vi "Flush Port.vi"(8 "error in (no error)":errorcluster, 10 "Port":T1="Mod6\\Port1", 11 "MPU in":refnum<class "MPU.lvclass">) -> (0 "error out":errorcluster, 3 "MPU out":refnum<class "MPU.lvclass">)   [LabVIEW 2018, in "Modbus_Processing_Unit.lvlib" / "MPU.lvclass"]
uses:
  MPU.lvclass
  PortType.ctl
  <vilib>/rvi/eio/common/nirviEmuTemplateMethod_errors.vi
  <vilib>/eio/EIOMethodNode/EIOMethodNode.xnode
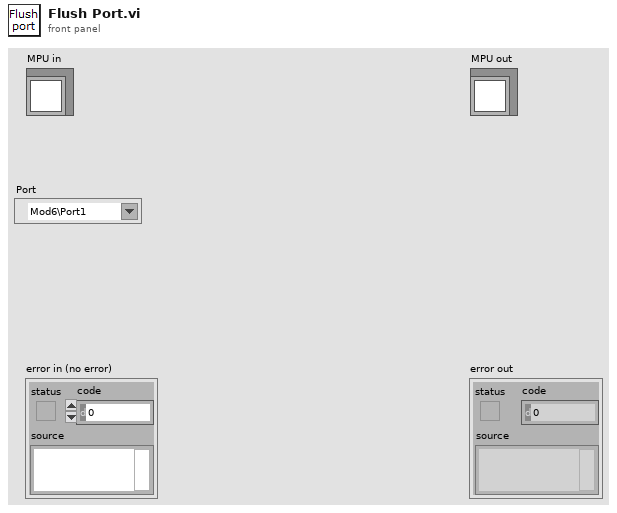
[diagram p1: front panel]
types:
  T1 = typedef "PortType.ctl" = refnum<k21>
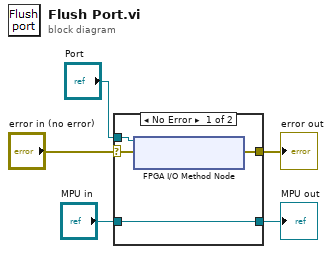
[diagram p0: block diagram]
diagram:
  n1 = case shown="No Error" "error in (no error)" {
    selector: "error in (no error)" -> [w7 w11]
    tunnel: [w8 w11] -> w4
    tunnel: [w9 w10] -> w2
    tunnel: "MPU in" -> [w9 w10]
    tunnel: "Port" -> [w6 _]
    frame No Error {
      n2 = xnode "FPGA I/O Method Node"("error in"=w7, "FPGA I/O In"=w6) -> ("error out"=w8:errorcluster)  [unwired: 1 out]
    }
    frame Error {
    }
  }
  "error out" <- w4
  "MPU out" <- w2
